vi "dfd_Render TF Item.vi"(0 "picture in":picture, 1 "fonts input":T3(array[cluster])=[{"Font Name:"="tahoma", "Size"=13, "Strikeout?"=FALSE, "Italic?"=FALSE, "Underline?"=FALSE, "Outline?"=TRUE, "Shadow?"=FALSE, "Bold?"=FALSE}, {"Font Name:"="tahoma", "Size"=13, "Strikeout?"=FALSE, "Italic?"=FALSE, "Underline?"=FALSE, "Outline?"=TRUE, "Shadow?"=FALSE, "Bold?"=FALSE}, {"Font Name:"="tahoma", "Size"=11, "Strikeout?"=FALSE, "Italic?"=FALSE, "Underline?"=FALSE, "Outline?"=TRUE, "Shadow?"=FALSE, "Bold?"=FALSE}], 2 "format coeffiecients":string="%#_g", 3 "variable":string="z", 5 "numerator":dbl[](array[numeric])=[1.0, 0.0, 0.0] format="%#_3g", 7 "denominator":dbl[](array[numeric])=[1.0] format="%#_3g", 9 "rect in":T1, 11 "delay":dbl, 12 "alignment(left, top)":T2, 13 "rendering options":T4={"coefficients ascending order"=FALSE, "render ascending order"=TRUE, "negative exponent"=TRUE, "add bracket"=FALSE}, 14 "equation type":enum16{"Continuous", "Discrete"}(ring)=enum."Discrete") -> (4 "picture out":picture, 6 "total rect":T1, 8 "polynomial":bool)   [LabVIEW 2017, in "NI_DigFilter_Process.lvlib"]
uses:
  <vilib>/addons/Digital Filter Design/NI_DigFilter_Process.lvlib
  <vilib>/Analysis/polynomials.llb/Remove Zero Coefficients (DBL).vi
  <vilib>/Analysis/NI_AALPro.lvlib
panel:
  in  "bar gap":u32
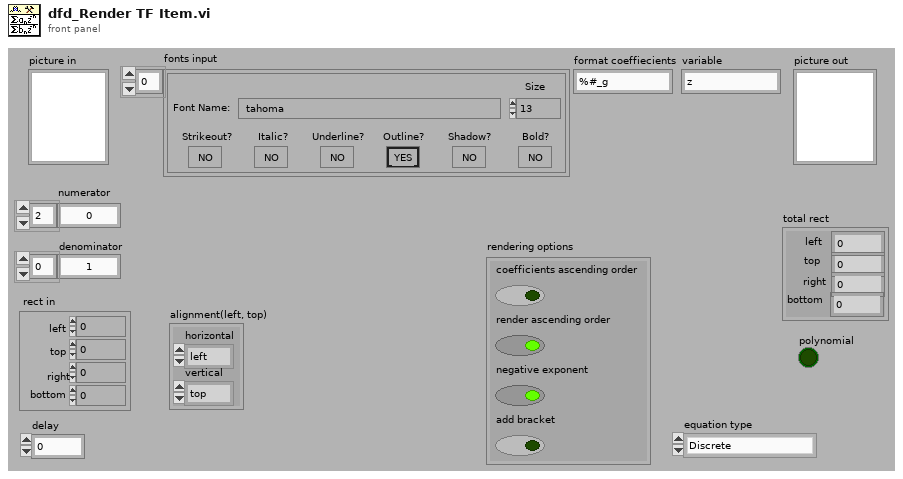
[diagram p1: front panel]
types:
  T1 = cluster{"left":i16, "top":i16, "right":i16, "bottom":i16}
  T2 = cluster{"horizontal":enum16{"left", "center", "right"}, "vertical":enum16{"top", "center", "bottom"}}
  T3 = cluster{"Font Name:":string, "Size":i16, "Strikeout?":bool, "Italic?":bool, "Underline?":bool, "Outline?":bool, "Shadow?":bool, "Bold?":bool}[]
  T4 = cluster{"coefficients ascending order":bool, "render ascending order":bool, "negative exponent":bool, "add bracket":bool}
  T5 = cluster{"coefficients ascending order":bool, "render ascending order":bool, "negative exponent":bool}
  T6 = cluster{"variable":string, cluster{"coefficients ascending order":bool, "render ascending order":bool, "negative exponent":bool}}
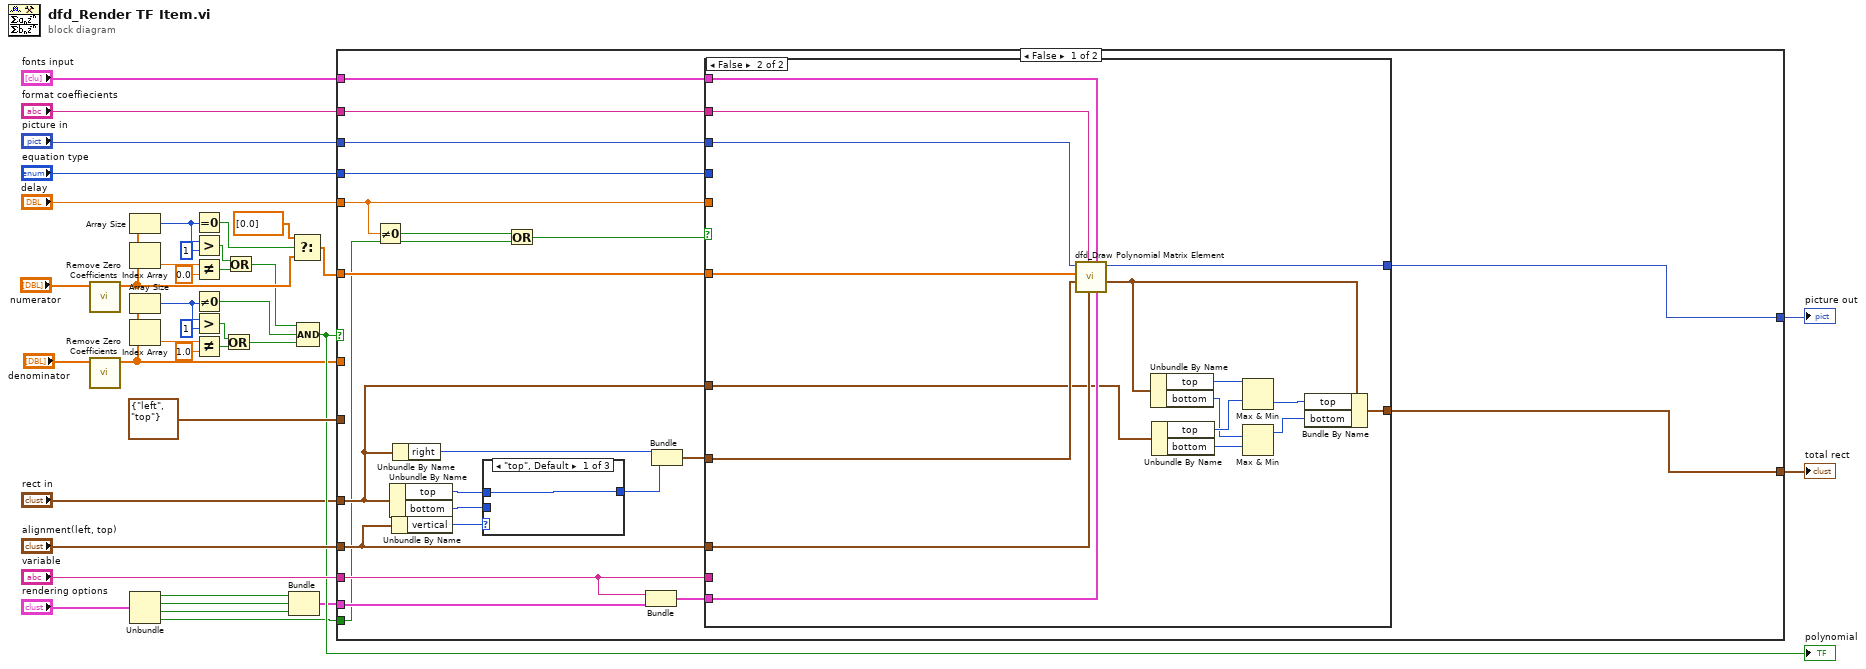
[diagram p0: block diagram]
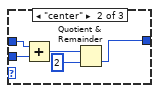
[diagram p2: hidden frame]
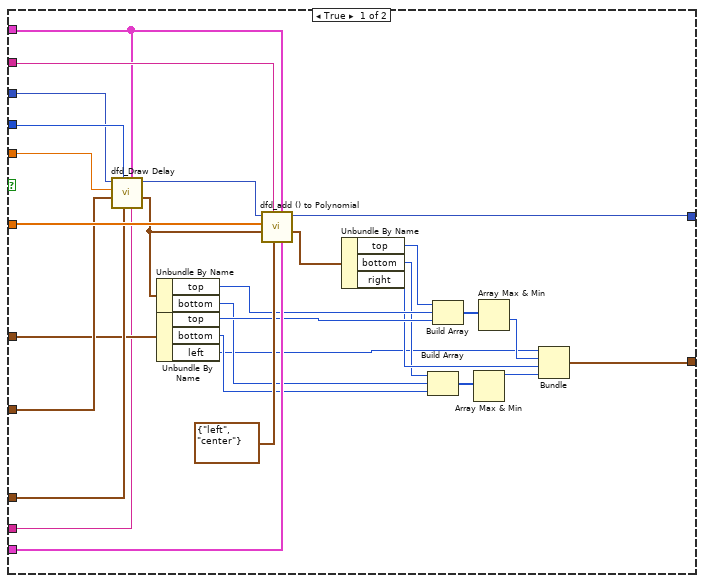
[diagram p4: hidden frame]
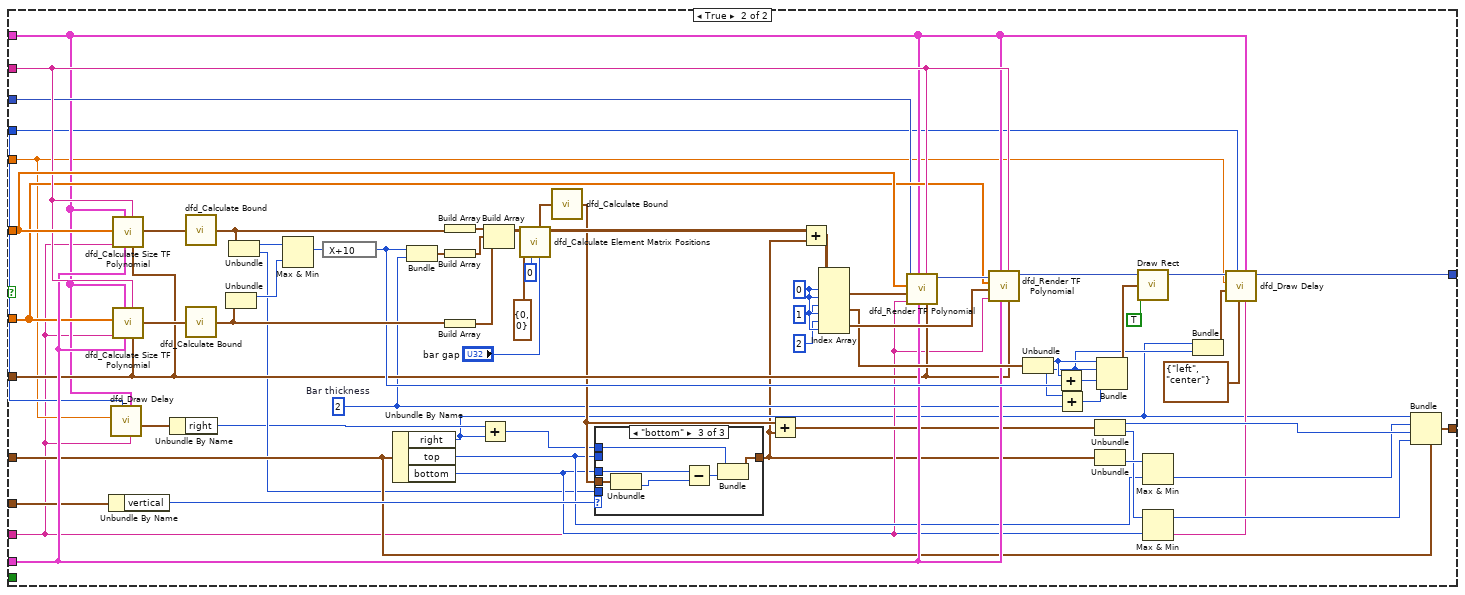
[diagram p5: hidden frame]
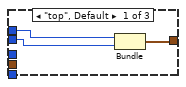
[diagram p6: hidden frame]
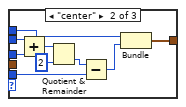
[diagram p7: hidden frame]
diagram:
  n1 = call-poly <vilib>:"Remove Zero Coefficients.vi"("P(x) In"="numerator") -> ("P(x) Out"=w15:dbl[])  [unwired: 2 in, 8 out]
  n2 = call-poly <vilib>:"Remove Zero Coefficients.vi"("P(x) In"="denominator") -> ("P(x) Out"=w26:dbl[])  [unwired: 2 in, 8 out]
  n3 = Array Size(array=w15) -> (size(s)=w17:i32)
  n4 = Index Array(array=w15) -> (element=w20:dbl)  [unwired: 1 in]
  n5 = Array Size(array=w26) -> (size(s)=w7:i32)
  n6 = Index Array(array=w26) -> (element=w24:dbl)  [unwired: 1 in]
  n7 = Unbundle("rendering options") -> ("coefficients ascending order"=w6:bool, "render ascending order"=w5:bool, "negative exponent"=w4:bool, "add bracket"=w1:bool)
  n8 = Equal To 0?(x=w17) -> (x = 0?=w16:bool)
  n9 = Greater?(x=w17, y=1) -> (0:w18:bool)
  n10 = Not Equal?(x=w20, y=0.0) -> (x != y?=w22:bool)
  n11 = Not Equal To 0?(x=w7) -> (x != 0?=w8:bool)
  n12 = Greater?(x=w7, y=1) -> (0:w12:bool)
  n13 = Not Equal?(x=w24, y=1.0) -> (x != y?=w11:bool)
  n14 = Or(x=w12, y=w11) -> (x .or. y?=w10:bool)
  n15 = Or(x=w18, y=w22) -> (x .or. y?=w9:bool)
  n16 = Bundle("coefficients ascending order"=w6, "render ascending order"=w5, "negative exponent"=w4) -> (w2:T5)  [unwired: 1 out]
  n17 = Select(t=dbl[] [0.0] ("P(x) Out"), s=w16, f=w15) -> (s? t:f=w14:dbl[])
  n18 = Compound Arithmetic op=AND(w9, w8, w10) -> (w32:bool)
  "polynomial" <- w32
  n19 = case shown="False" w32 {
    tunnel: w14 -> [w58 w179]
    tunnel: "format coeffiecients" -> [w60 w178]
    tunnel: w2 -> [w44 w154]
    tunnel: "fonts input" -> [w61 w124]
    tunnel: w26 -> [_ w151]
    tunnel: [w62 w144] -> w38
    tunnel: [w57 w127] -> w37
    tunnel: "variable" -> [w45 w121]
    tunnel: "alignment(left, top)" -> [w49 w149]
    tunnel: "rect in" -> [w47 w128]
    tunnel: T2 {"horizontal"=enum."left", "vertical"=enum."top"} ("alignment(left, top)") -> [_ w147]
    tunnel: "picture in" -> [w59 w146]
    tunnel: "delay" -> [w55 w122]
    tunnel: "equation type" -> [w56 w123]
    tunnel: w1 -> [w43 _]
    frame False {
      n20 = Not Equal To 0?(x=w55) -> (x != 0?=w42:bool)
      n21 = Unbundle By Name(w47) -> ("top"=w51:i16, "bottom"=w52:i16)
      n22 = Unbundle By Name(w49) -> ("vertical"=w50:enum16{"top", "center", "bottom"})
      n23 = Unbundle By Name(w47) -> ("right"=w53:i16)
      n24 = case shown="\"top\", Default" w50 {
        tunnel: w51 -> [w63 w68 _]
        tunnel: w52 -> [_ w67 w69]
        tunnel: [w63 w64 w69] -> w54
        frame "top", Default {
        }
        frame "center" {
          n25 = Add(x=w68, y=w67) -> (x+y=w66:i16)
          n26 = Quotient & Remainder(x=w66, y=i16 2) -> (floor(x/y)=w64:i16)  [unwired: 1 out]
        }
        frame "bottom" {
        }
      }
      n27 = Or(x=w42, y=w43) -> (x .or. y?=w41:bool)
      n28 = Bundle("variable"=w45, w44) -> (w46:T6)  [unwired: 1 out]
      n29 = Bundle("right"=w53, "bottom"=w54) -> (w48:cluster{"right":i16, "bottom":i16})  [unwired: 1 out]
      n30 = case shown="False" w41 {
        tunnel: [w88 w115] -> w62
        tunnel: w61 -> [w95 w114]
        tunnel: w60 -> [w98 w113]
        tunnel: w59 -> [w93 w112]
        tunnel: w58 -> [w97 w111]
        tunnel: [w71 w105] -> w57
        tunnel: w49 -> [w91 w110]
        tunnel: w56 -> [w96 _]
        tunnel: w55 -> [w94 _]
        tunnel: w48 -> [w90 w109]
        tunnel: w47 -> [w85 w107]
        tunnel: w46 -> [w84 w108]
        tunnel: w45 -> [w70 _]
        frame True {
          n31 = call <vilib>:"dfd_Draw Delay.vi"("variable"=w70, "fonts input"=w95, "alignment(left, top)"=w91, "equation type"=w96, "origin"=w90, "delay"=w94, "picture"=w93) -> ("text rect"=w87:T1, "new picture"=w92:picture)  [unwired: 3 out]
          n32 = Unbundle By Name(w87) -> ("top"=w82:i16, "bottom"=w75:i16)
          n33 = Unbundle By Name(w85) -> ("top"=w81:i16, "bottom"=w74:i16, "left"=w72:i16)
          n34 = call <vilib>:"dfd_add () to Polynomial.vi"("format control"=w84, "fonts input"=w95, "alignment(left, top)"=T2 {"horizontal"=enum."left", "vertical"=enum."center"}, "format string"=w98, "rect in"=w87, "polynomial"=w97, "picture in"=w92) -> ("rect out"=w86:T1, "new picture"=w88:picture)  [unwired: 3 out]
          n35 = Unbundle By Name(w86) -> ("top"=w83:i16, "bottom"=w76:i16, "right"=w78:i16)
          n36 = Build Array(w76, w75, w74) -> (w77:i16[])
          n37 = Build Array(w83, w82, w81) -> (w80:i16[])
          n38 = Array Max & Min(array=w77) -> (max value=w73:i16)  [unwired: 3 out]
          n39 = Array Max & Min(array=w80) -> (min value=w79:i16)  [unwired: 3 out]
          n40 = Bundle("left"=w72, w79, "right"=w78, w73) -> (w71:cluster{"left":i16, i16, "right":i16, i16})  [unwired: 1 out]
        }
        frame False {
          n41 = call <vilib>:"dfd_Draw Polynomial Matrix Element.vi"("format control"=w108, "fonts input"=w114, "alignment(left, top)"=w110, "format string"=w113, "origin"=w109, "coefficients"=w111, "picture in"=w112) -> ("location"=w106:T1, "picture out"=w115:picture)  [unwired: 3 out]
          n42 = Unbundle By Name(w106) -> ("top"=w104:i16, "bottom"=w102:i16)
          n43 = Unbundle By Name(w107) -> ("top"=w103:i16, "bottom"=w101:i16)
          n44 = Max & Min(x=w104, y=w103) -> (min(x,y)=w100:i16)  [unwired: 1 out]
          n45 = Max & Min(x=w102, y=w101) -> (max(x,y)=w99:i16)  [unwired: 1 out]
          n46 = Bundle By Name(cluster=w106, "top"=w100, "bottom"=w99) -> (w105:T1)
        }
      }
    }
    frame True {
      w167 = 0 ("index (row)")
      w126 = 2  # Bar thickness
      n47 = Unbundle By Name(w149) -> ("vertical"=w137:enum16{"top", "center", "bottom"})
      n48 = call <vilib>:"dfd_Draw Delay.vi"("variable"=w121, "fonts input"=w124, "equation type"=w123, "delay"=w122) -> ("text rect"=w120:T1)  [unwired: 3 in, 4 out]
      n49 = call <vilib>:"dfd_Calculate Size TF Polynomial.vi"("alignment(left, top)"=w147, "format string"=w178, "rendering options"=w154, "Fonts Input"=w124, "variable"=w121, "coefficients"=w179) -> ("text rect"=w181:T1)  [unwired: 1 in, 4 out]
      n50 = call <vilib>:"dfd_Calculate Size TF Polynomial.vi"("alignment(left, top)"=w147, "format string"=w178, "rendering options"=w154, "Fonts Input"=w124, "variable"=w121, "coefficients"=w151) -> ("text rect"=w182:T1)  [unwired: 1 in, 4 out]
      n51 = Unbundle By Name(w120) -> ("right"=w119:i16)
      n52 = call <vilib>:"dfd_Calculate Bound.vi"("rect"=w181) -> ("Bounds"=w171:cluster{"Width":i16, "Height":i16})
      n53 = call <vilib>:"dfd_Calculate Bound.vi"("rect"=w182) -> ("Bounds"=w174:cluster{"Width":i16, "Height":i16})
      n54 = Unbundle(w174) -> ("Width"=w173:i16)  [unwired: 1 out]
      n55 = Unbundle(w171) -> ("Width"=w148:i16, "Height"=w125:i16)
      n56 = Max & Min(x=w148, y=w173) -> (max(x,y)=w159:i16)  [unwired: 1 out]
      n57 = expression code="X+10"(w159) -> (w155:i16)
      n58 = Unbundle By Name(w128) -> ("right"=w117:i16, "top"=w130:i16, "bottom"=w129:i16)
      n59 = Bundle(w155, "Bar thickness"=w126) -> (w170:cluster{i16, "Bar thickness":i32})  [unwired: 1 out]
      n60 = Build Array(w171) -> (w177:cluster{"Width":i16, "Height":i16}[])
      n61 = Build Array(w170) -> (w172:cluster{i16, "Bar thickness":i32}[])
      n62 = Build Array(w174) -> (w176:cluster{"Width":i16, "Height":i16}[])
      n63 = Add(x=w119, y=w117) -> (x+y=w118:i16)
      n64 = Build Array(w177, w172, w176) -> (w175:cluster{"Width":i16, "Bar thickness":i32}[][])
      n65 = call <vilib>:"dfd_Calculate Element Matrix Positions.vi"("Height Gap"="bar gap", "Width Gap"=u32 0, "origin"=cluster{"x":i16, "y":i16} {"x"=0, "y"=0}, "Object Bounds"=w175) -> ("Origins Position"=w168:cluster{"x":i16, "y":i16}[][], "rect"=w169:T1)  [unwired: 2 in, 4 out]
      n66 = call <vilib>:"dfd_Calculate Bound.vi"("rect"=w169) -> ("Bounds"=w138:cluster{"Width":i16, "Height":i16})
      n67 = case shown="\"bottom\"" w137 {
        tunnel: [w185 w187 w198] -> w116
        tunnel: w125 -> [_ w186 _]
        tunnel: w138 -> [_ _ w200]
        tunnel: w118 -> [w184 w188 w196]
        tunnel: w130 -> [w183 w194 _]
        tunnel: w129 -> [_ w193 w197]
        frame "top", Default {
          n68 = Bundle(w184, "top"=w183) -> (w185:cluster{i16, "top":i16})  [unwired: 1 out]
        }
        frame "center" {
          n69 = Add(x=w194, y=w193) -> (x+y=w192:i16)
          n70 = Quotient & Remainder(x=w192, y=i16 2) -> (floor(x/y)=w190:i16)  [unwired: 1 out]
          n71 = Subtract(x=w190, y=w186) -> (x-y=w189:i16)
          n72 = Bundle(w188, w189) -> (w187:cluster{i16, i16})  [unwired: 1 out]
        }
        frame "bottom" {
          n73 = Unbundle(w200) -> ("Height"=w195:i16)  [unwired: 1 out]
          n74 = Subtract(x=w197, y=w195) -> (x-y=w199:i16)
          n75 = Bundle(w196, w199) -> (w198:cluster{i16, i16})  [unwired: 1 out]
        }
      }
      n76 = Add(x=w138, y=w116) -> (x+y=w131:cluster{i16, i16})
      n77 = Add(x=w168, y=w116) -> (x+y=w162:cluster{i16, i16}[][])
      n78 = Index Array(array=w162, index (row) #1=w167, index (col) #1=w167, index (row) #2=1 ("disabled index (row)"), index (col) #2=w167, index (row) #3=2 ("disabled index (row)"), index (col) #3=w167) -> (element #1=w164:cluster{i16, i16}, element #2=w161:cluster{i16, i16}, element #3=w163:cluster{i16, i16})
      n79 = call <vilib>:"dfd_Render TF Polynomial.vi"("alignment(left, top)"=w147, "format string"=w178, "rendering options"=w154, "Fonts Input"=w124, "variable"=w121, "origin"=w164, "coefficients"=w179, "picture in"=w146) -> ("rendered equation"=w180:picture)  [unwired: 3 out]
      n80 = call <vilib>:"dfd_Render TF Polynomial.vi"("alignment(left, top)"=w147, "format string"=w178, "rendering options"=w154, "Fonts Input"=w124, "variable"=w121, "origin"=w163, "coefficients"=w151, "picture in"=w180) -> ("rendered equation"=w150:picture)  [unwired: 3 out]
      n81 = Unbundle(w161) -> (w160:i16, w143:i16)
      n82 = Add(x=w160, y=w155) -> (x+y=w142:i16)
      n83 = Add(x=w143, y=w126) -> (x+y=w158:i32)
      n84 = Unbundle(w131) -> (w136:i16, w134:i16)
      n85 = Unbundle(w116) -> ("top"=w135:i16)  [unwired: 1 out]
      n86 = Bundle(w160, w143, w142, w158) -> (w157:cluster{i16, i16, i16, i32})  [unwired: 1 out]
      n87 = call <vilib>:"Draw Rect.vi"("picture"=w150, "rect"=w157, "fill?(F)"=TRUE) -> ("new picture"=w145:picture)  [unwired: 2 in, 4 out]
      n88 = Max & Min(x=w135, y=w130) -> (min(x,y)=w133:i16)  [unwired: 1 out]
      n89 = Max & Min(x=w134, y=w129) -> (max(x,y)=w132:i16)  [unwired: 1 out]
      n90 = Bundle("right"=w117, w143) -> (w141:cluster{"right":i16, i16})  [unwired: 1 out]
      n91 = call <vilib>:"dfd_Draw Delay.vi"("variable"=w121, "fonts input"=w124, "alignment(left, top)"=T2 {"horizontal"=enum."left", "vertical"=enum."center"}, "equation type"=w123, "origin"=w141, "delay"=w122, "picture"=w145) -> ("new picture"=w144:picture)  [unwired: 4 out]
      n92 = Bundle(cluster=w128, "left"=w117, "top"=w133, "right"=w136, "bottom"=w132) -> (w127:T1)
    }
  }
  "picture out" <- w38
  "total rect" <- w37
